vi "sailingPoints.vi"(9 "Mission Notifiers":T1, 10 "NotifierReff":T2, 11 "Waypoint queue":refnum<queue>) -> (0 "Number of sailing points added":i32, 1 "Added sailing points?":bool, 2 "Added intermediate point?":bool, 3 "Waypoint queue out":refnum<queue>)   [LabVIEW 2013]
doc: "If next waypoint is not within irons range, go to it. \nIf it is in irons range, [add code that will deal with it]\n\n3/17/2014 -Kaitlin"
uses:
  Classes/Waypoint/Waypoint.lvclass
  Data/TypeDefs/Notifiers.ctl
  Data/TypeDefs/UTM Location.ctl
  Data/TypeDefs/Sail Set Suggestions.ctl
  Data/TypeDefs/Rudder Set Suggestions.ctl
  Data/TypeDefs/OverrideInformation.ctl
  Data/TypeDefs/OverrideMode.ctl
  Data/TypeDefs/MotorSetup.ctl
  Data/TypeDefs/DynamixelSetupInfo.ctl
  Data/TypeDefs/AirmarStatus.ctl
  Data/TypeDefs/HardwareOnline.ctl
  Data/TypeDefs/DynamixelCycleTracker.ctl
  Data/TypeDefs/RC Input Values.ctl
  Data/TypeDefs/MissionNotifiers.ctl
  Classes/Missions/GenericMission/GenericMission.lvclass
  Classes/Obstacle/Obstacle.lvclass
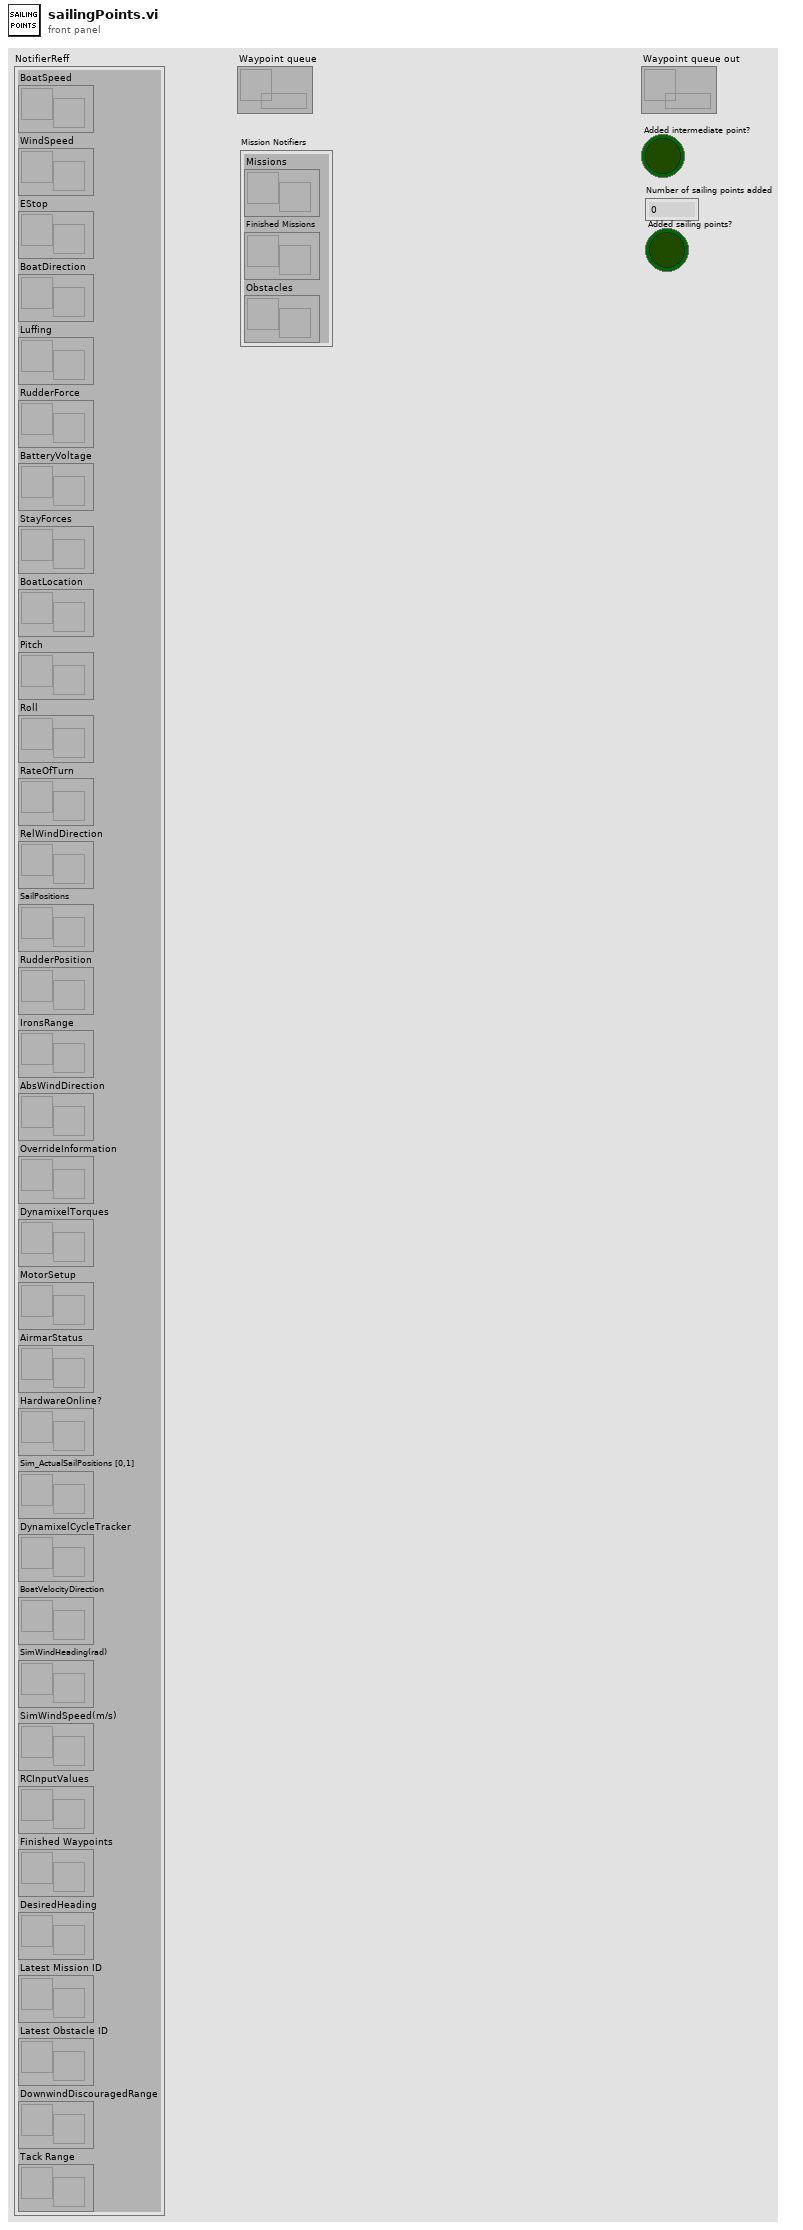
[diagram p1: front panel]
types:
  T1 = typedef "MissionNotifiers.ctl" = cluster{"Missions":refnum<notifier>, "Finished Missions":refnum<notifier>, "Obstacles":refnum<notifier>}
  T2 = typedef "Notifiers.ctl" = cluster{"BoatSpeed":refnum<notifier>, "WindSpeed":refnum<notifier>, "EStop":refnum<notifier>, "BoatDirection":refnum<notifier>, "Luffing":refnum<notifier>, "RudderForce":refnum<notifier>, "BatteryVoltage":refnum<notifier>, "StayForces":refnum<notifier>, "BoatLocation":refnum<notifier>, "Pitch":refnum<notifier>, "Roll":refnum<notifier>, "RateOfTurn":refnum<notifier>, "RelWindDirection":refnum<notifier>, "SailPositions":refnum<notifier>, "RudderPosition":refnum<notifier>, "IronsRange":refnum<notifier>, "AbsWindDirection":refnum<notifier>, "OverrideInformation":refnum<notifier>, "DynamixelTorques":refnum<notifier>, "MotorSetup":refnum<notifier>, "AirmarStatus":refnum<notifier>, "HardwareOnline?":refnum<notifier>, "Sim_ActualSailPositions [0,1]":refnum<notifier>, "DynamixelCycleTracker":refnum<notifier>, "BoatVelocityDirection":refnum<notifier>, "SimWindHeading(rad)":refnum<notifier>, "SimWindSpeed(m/s)":refnum<notifier>, "RCInputValues":refnum<notifier>, "Finished Waypoints":refnum<notifier>, "DesiredHeading":refnum<notifier>, "Latest Mission ID":refnum<notifier>, "Latest Obstacle ID":refnum<notifier>, "DownwindDiscouragedRange":refnum<notifier>, "Tack Range":refnum<notifier>}
  T3 = typedef "UTM Location.ctl" = cluster{"UTM Zone":dbl, "Hemisphere":enum16{"North", "South"}, "East":dbl, "North":dbl}
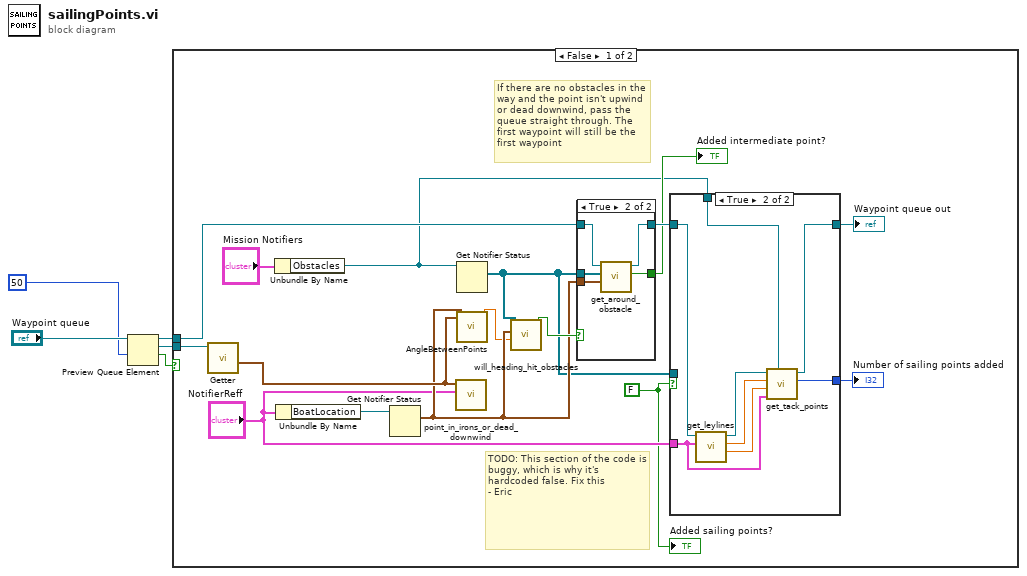
[diagram p0: block diagram]
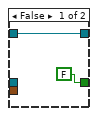
[diagram p2: hidden frame]
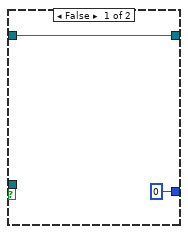
[diagram p3: hidden frame]
diagram:
  n1 = Preview Queue Element(queue="Waypoint queue", timeout in ms (-1)=50) -> (queue out=w4:refnum<queue>, element=w3:refnum<class "Waypoint.lvclass">, timed out?=w1:bool)  [unwired: 1 in, 1 out]
  n2 = case shown="False" w1 {
    tunnel: w4 -> [w12 _]
    tunnel: w3 -> [w11 _]
    frame False {
      w6 = FALSE
      # "TODO: This section of the code is buggy, which is why it's hardcoded false. Fix this\n- Eric"
      # "If there are no obstacles in the way and the point isn't upwind or dead downwind, pass the queue straight through. The first waypoint will still be the first waypoint"
      n3 = call "Getter.vi"("Waypoint In"=w11) -> ("Coords"=w18:T3)  [unwired: 6 in, 4 out]
      n4 = Unbundle By Name("Mission Notifiers") -> ("Obstacles"=w8:refnum<notifier>)
      n5 = Unbundle By Name("NotifierReff") -> ("BoatLocation"=w21:refnum<notifier>)
      n6 = Get Notifier Status(notifier=w21) -> (current notification=w15:T3)  [unwired: 1 in, 4 out]
      n7 = call "point_in_irons_or_dead_downwind.vi"("NotifierReff"="NotifierReff", "Point"=w18) -> ()  [unwired: 7 in, 3 out]
      n8 = Get Notifier Status(notifier=w8) -> (current notification=w9:refnum<class "Obstacle.lvclass">[])  [unwired: 1 in, 4 out]
      n9 = call "AngleBetweenPoints.vi"("Point 2"=w18, "Point 1"=w15) -> ("Angle from P1 to P2"=w14:dbl)  [unwired: 9 in]
      n10 = call "will_heading_hit_obstacles.vi"("Heading"=w14, "Boat Location"=w15, "Obstacle array"=w9) -> ("Will boat hit any obstacles?"=w17:bool)  [unwired: 8 in]
      n11 = case shown="True" w17 {
        tunnel: w12 -> [w23 w28]
        tunnel: [w23 w24] -> w16
        tunnel: w9 -> [_ w27]
        tunnel: w15 -> [_ w26]
        tunnel: [FALSE ("Added intermediate point?") w25] -> w13
        frame False {
        }
        frame True {
          n12 = call "get_around_obstacle.vi"("Boat location"=w26, "Obstacle array"=w27, "Waypoint queue"=w28) -> ("Added intermediate point?"=w25:bool, "Waypoint queue out"=w24:refnum<queue>)  [unwired: 7 in]
        }
      }
      "Added intermediate point?" <- w13
      n13 = case shown="True" w6 {
        tunnel: w16 -> [w30 w38]
        tunnel: [w30 w32] -> w20
        tunnel: "NotifierReff" -> [_ w34]
        tunnel: w9 -> [_ _]
        tunnel: w8 -> [_ w33]
        tunnel: [0 ("Number of sailing points added") w31] -> w7
        frame False {
        }
        frame True {
          n14 = call "get_leylines.vi"("NotifierReff"=w34, "Waypoint queue"=w38) -> ("Other leyline"=w35:dbl, "Final leyline"=w36:dbl, "Waypoint queue out"=w37:refnum<queue>)  [unwired: 7 in]
          n15 = call "get_tack_points.vi"("Obstacle Notifier"=w33, "NotifierReff"=w34, "Other leyline (deg)"=w35, "Final leyline (deg)"=w36, "Waypoint queue"=w37) -> ("Number of sailing points added"=w31:i32, "Waypoint queue OUT"=w32:refnum<queue>)  [unwired: 5 in]
        }
      }
      "Waypoint queue out" <- w20
      "Number of sailing points added" <- w7
      "Added sailing points?" <- w6
    }
    frame True {
    }
  }
